vi "Get Printer.vi"(8 "error in (no error)":errorcluster caption="entrée d'erreur (pas d'erreur)", 11 "Class Printer (Default) en entrée":refnum<class "Class Printer (Default).lvclass">) -> (0 "error out":errorcluster caption="sortie d'erreur", 2 "Printer":string, 3 "Class Printer (Default) en sortie":refnum<class "Class Printer (Default).lvclass">)   [LabVIEW 2020, in "Library Instrument & Equipement.lvlib" / "Library Printer.lvlib" / "Class Printer (Default).lvclass"]
uses:
  Class Printer (Default).lvclass
  Class Printer (Default).lvclass/Class Printer (Default).ctl
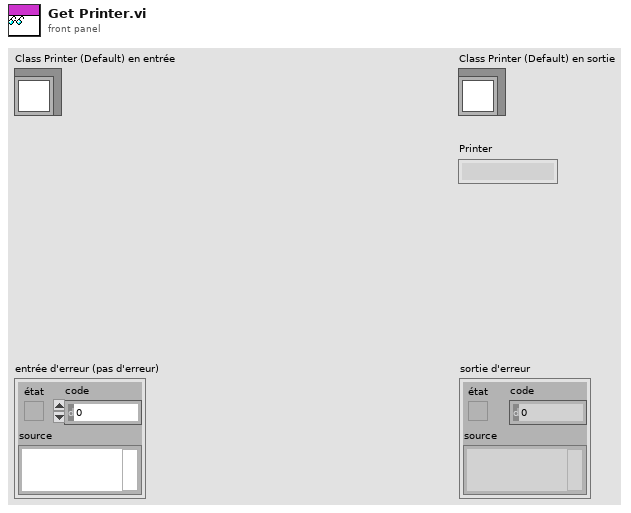
[diagram p1: front panel]
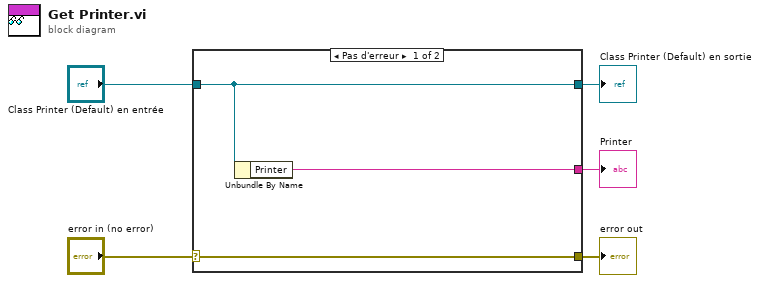
[diagram p0: block diagram]
diagram:
  n1 = case shown="Pas d'erreur" "error in (no error)" {
    selector: "error in (no error)" -> [w8 w9]
    tunnel: [w8 w9] -> w4
    tunnel: [w7 w10] -> w2
    tunnel: "Class Printer (Default) en entrée" -> [w7 w10]
    tunnel: [w6 _] -> w1
    frame No Error {
      n2 = Unbundle By Name(w7) -> ("Printer"=w6:string)
    }
    frame Error {
    }
  }
  "error out" <- w4
  "Class Printer (Default) en sortie" <- w2
  "Printer" <- w1
